vi "顺启灯.vi"() -> ()   [LabVIEW 2018]
panel:
  in  "停止":bool
  in  "速度":dbl(slide) scale=0.0..3000.0
  out "布尔 7":bool
  out "布尔 6":bool
  out "布尔 5":bool
  out "布尔 4":bool
  out "布尔 3":bool
  out "布尔 2":bool
  out "布尔":bool
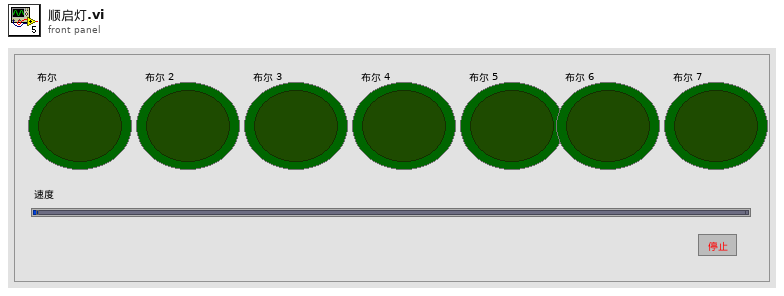
[diagram p1: front panel]
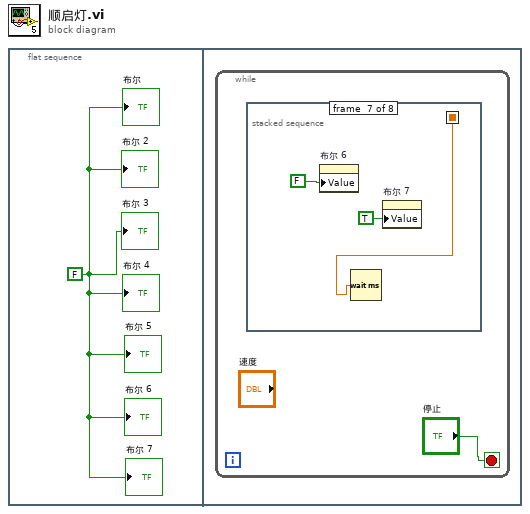
[diagram p0: block diagram]
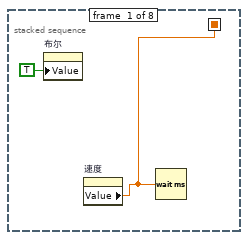
[diagram p2: hidden frame]
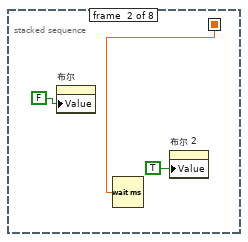
[diagram p3: hidden frame]
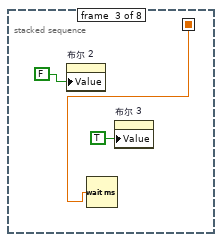
[diagram p4: hidden frame]
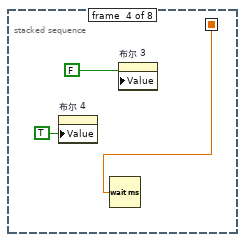
[diagram p5: hidden frame]
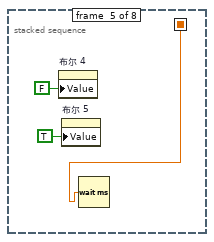
[diagram p6: hidden frame]
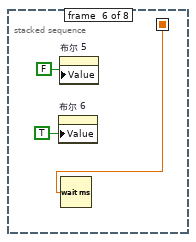
[diagram p7: hidden frame]
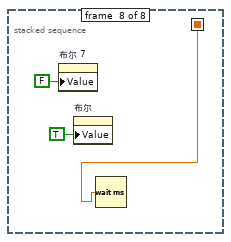
[diagram p8: hidden frame]
diagram:
  n1 = flat-sequence {
    frame #0 {
      w1 = FALSE
      "布尔" <- w1
      "布尔 2" <- w1
      "布尔 3" <- w1
      "布尔 4" <- w1
      "布尔 5" <- w1
      "布尔 6" <- w1
      "布尔 7" <- w1
    }
    frame #1 {
      n2 = while {
        stop <- "停止" stop-if-true
        n3 = stacked-sequence {
          seq-local: [w3 _ _ _ _ _ _ _] -> [_ w7 w10 w13 w16 w19 w22 w25]
          frame #0 {
            n4 = property on="布尔" class="Bool (严格)"("Value"=TRUE ("布尔")) -> ()  [unwired: 2 in, 2 out]
            n5 = property on="速度" class="Slide (严格)"() -> ("Value"=w3:dbl)  [unwired: 2 in, 2 out]
            n6 = Wait (ms)(milliseconds to wait=w3) -> ()  [unwired: 1 out]
          }
          frame #1 {
            n7 = property on="布尔" class="Bool (严格)"("Value"=FALSE ("布尔")) -> ()  [unwired: 2 in, 2 out]
            n8 = Wait (ms)(milliseconds to wait=w7) -> ()  [unwired: 1 out]
            n9 = property on="布尔 2" class="Bool (严格)"("Value"=TRUE ("布尔 2")) -> ()  [unwired: 2 in, 2 out]
          }
          frame #2 {
            n10 = property on="布尔 2" class="Bool (严格)"("Value"=FALSE ("布尔 2")) -> ()  [unwired: 2 in, 2 out]
            n11 = Wait (ms)(milliseconds to wait=w10) -> ()  [unwired: 1 out]
            n12 = property on="布尔 3" class="Bool (严格)"("Value"=TRUE ("布尔 3")) -> ()  [unwired: 2 in, 2 out]
          }
          frame #3 {
            n13 = property on="布尔 4" class="Bool (严格)"("Value"=TRUE ("布尔 4")) -> ()  [unwired: 2 in, 2 out]
            n14 = Wait (ms)(milliseconds to wait=w13) -> ()  [unwired: 1 out]
            n15 = property on="布尔 3" class="Bool (严格)"("Value"=FALSE ("布尔 3")) -> ()  [unwired: 2 in, 2 out]
          }
          frame #4 {
            n16 = property on="布尔 4" class="Bool (严格)"("Value"=FALSE ("布尔 4")) -> ()  [unwired: 2 in, 2 out]
            n17 = property on="布尔 5" class="Bool (严格)"("Value"=TRUE ("布尔 5")) -> ()  [unwired: 2 in, 2 out]
            n18 = Wait (ms)(milliseconds to wait=w16) -> ()  [unwired: 1 out]
          }
          frame #5 {
            n19 = property on="布尔 6" class="Bool (严格)"("Value"=TRUE ("布尔 6")) -> ()  [unwired: 2 in, 2 out]
            n20 = property on="布尔 5" class="Bool (严格)"("Value"=FALSE ("布尔 5")) -> ()  [unwired: 2 in, 2 out]
            n21 = Wait (ms)(milliseconds to wait=w19) -> ()  [unwired: 1 out]
          }
          frame #6 {
            n22 = property on="布尔 6" class="Bool (严格)"("Value"=FALSE ("布尔 6")) -> ()  [unwired: 2 in, 2 out]
            n23 = Wait (ms)(milliseconds to wait=w22) -> ()  [unwired: 1 out]
            n24 = property on="布尔 7" class="Bool (严格)"("Value"=TRUE ("布尔 7")) -> ()  [unwired: 2 in, 2 out]
          }
          frame #7 {
            n25 = property on="布尔 7" class="Bool (严格)"("Value"=FALSE ("布尔 7")) -> ()  [unwired: 2 in, 2 out]
            n26 = property on="布尔" class="Bool (严格)"("Value"=TRUE ("布尔")) -> ()  [unwired: 2 in, 2 out]
            n27 = Wait (ms)(milliseconds to wait=w25) -> ()  [unwired: 1 out]
          }
        }
      }
    }
  }
